vi "test_mode_selector.vi"(10 "test mode":string[](array[string])) -> (2 "test mode":T1)   [LabVIEW 2015]
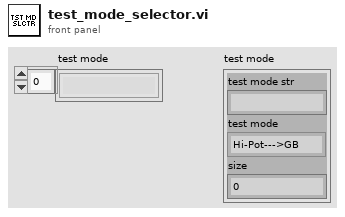
[diagram p1: front panel]
types:
  T1 = cluster{"test mode str":string, "test mode":enum16{"Hi-Pot--->GB", "GB--->Hi-Pot", "Hi-Pot only", "GB only"}, "size":i32}
  T2 = enum16{"Hi-Pot--->GB", "GB--->Hi-Pot", "Hi-Pot only", "GB only"}
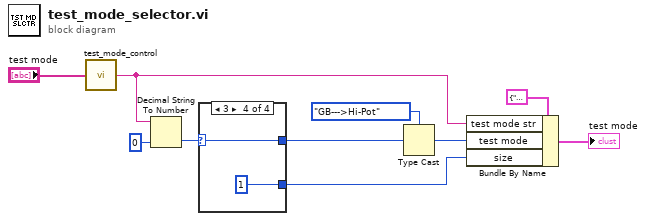
[diagram p0: block diagram]
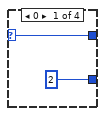
[diagram p2: hidden frame]
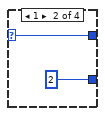
[diagram p3: hidden frame]
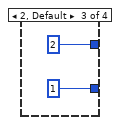
[diagram p4: hidden frame]
diagram:
  n1 = call "test_mode_control.vi"("test mode"="test mode") -> ("test mode str out"=w5:string)  [unwired: 6 in]
  n2 = Decimal String To Number(string=w5, default (0L)=u16 0 ("default (0 I32)")) -> (number=w9:u16)  [unwired: 1 in, 1 out]
  n3 = case shown="3" w9 {
    selector: w9 -> [w12 w14 _ w18]
    tunnel: [w12 w14 u16 2 w18] -> w10
    tunnel: [2 2 1 1] -> w3
    frame 0 {
    }
    frame 1 {
    }
    frame 2, Default {
    }
    frame 3 {
    }
  }
  n4 = Type Cast(type=T2."GB--->Hi-Pot", x=w10) -> (*(type *) &x=w4:T2)
  n5 = Bundle By Name(cluster=T1 {"test mode str"="", "test mode"=enum."Hi-Pot only", "size"=0} ("test mode"), "test mode str"=w5, "test mode"=w4, "size"=w3) -> (→"test mode":T1)
